vi "Build Control Reference Map.vi"(8 "error in (no error)":errorcluster, 11 "Control Refs":refnum<vi>[](array[refnum])) -> (0 "error out":errorcluster, 3 "Control Ref Map":map{string, refnum<vi>}(c390))   [LabVIEW 2020, in "MacroAssert.lvlib"]
doc: "Builds a map of label-reference pairs from <B>Control Refs</B>."
uses:
  MacroAssert.lvlib
  <vilib>/Utility/error.llb/Error Cluster From Error Code.vi
  SubVIs/Custom Errors/Custom Errors.lvlib
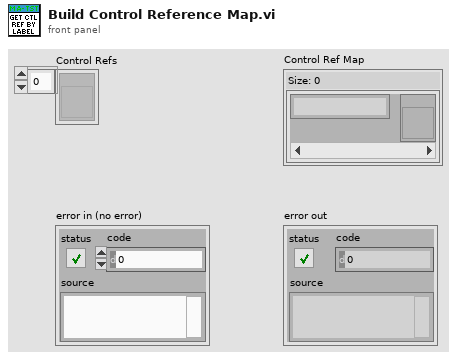
[diagram p1: front panel]
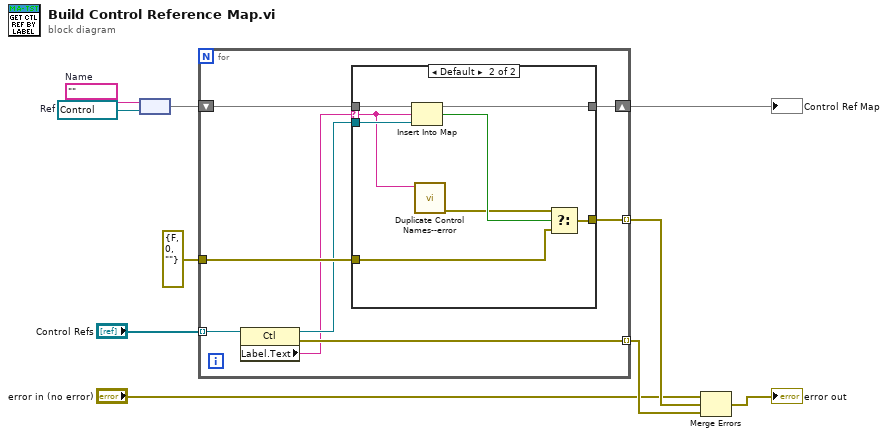
[diagram p0: block diagram]
diagram:
  w4 = ""  # Name
  w5 = refnum<vi> refnum  # Ref
  n1 = node(w4, w5) -> (w3:map{string, refnum<vi>})
  n2 = for {
    tunnel: "Control Refs" -> [w17] mode=indexing
    tunnel: [w16] -> w9 mode=indexing
    shift-right: [w13] -> w2
    shift-left: w3 -> [w15]
    tunnel: [w11] -> w10 mode=indexing
    tunnel: errorcluster {"status"=FALSE, "code"=0, "source"=""} ("error in (no error)") -> [w18]
    n3 = property class="Ctl"(reference=w17) -> (reference out=w14:refnum<vi>, error out=w16:errorcluster, "Label.Text"=w12:string)  [unwired: 1 in]
    n4 = case shown="Default" w12 {
      selector: w12 -> [_ w25]
      tunnel: w15 -> [w20 w28]
      tunnel: w14 -> [_ w27]
      tunnel: [w20 w26] -> w13
      tunnel: [w19 w22] -> w11
      tunnel: w18 -> [w19 w21]
      frame "error in (no error)", "error out" {
        # "exclude these from map"
      }
      frame Default {
        n5 = Insert Into Map(map in=w28, key=w25, value=w27) -> (map out=w26:map{string, refnum<vi>}, key already included?=w24:bool)  [unwired: 1 out]
        n6 = call "Duplicate Control Names--error.vi"("Control Name"=w25) -> ("error out"=w23:errorcluster)  [unwired: 10 in]
        n7 = Select(t=w23, s=w24, f=w21) -> (s? t:f=w22:errorcluster)
      }
    }
  }
  "Control Ref Map" <- w2
  n8 = Merge Errors("error in (no error)", w10, w9) -> (→"error out":errorcluster)
